vi "dNetOut_dOutH1.vi"(11 "OutH2":sgl[](array[numeric])) -> (3 "Output":sgl[](array[numeric]))   [LabVIEW 2020]
uses:
  <vilib>/rvi/Memory/Memory_Emulation/nirvimemoryFastEmulation.vi
  <vilib>/rvi/Memory/Memory_Emulation/nirvimemoryEmulation.vi
  <vilib>/rvi/Emulation/niFpgaEmulationIsFPGAContextNoSignature.vi
  <vilib>/rvi/DataTransferAndStorage/Container/Common/niFpgaContainerGetUniqueNameForEmu.vi
  <vilib>/rvi/Emulation/niFpgaProcessEmulError.vi
  <vilib>/rvi/Emulation/niFpgaSctlEmulationGetInTimedLoop.vi
  <vilib>/rvi/errors/nirviReportUnexpectedCaseInternalError (U32).vi
  <vilib>/rvi/DataTransferAndStorage/Container/XNode/niFpgaContainer.xnode
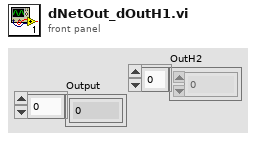
[diagram p1: front panel]
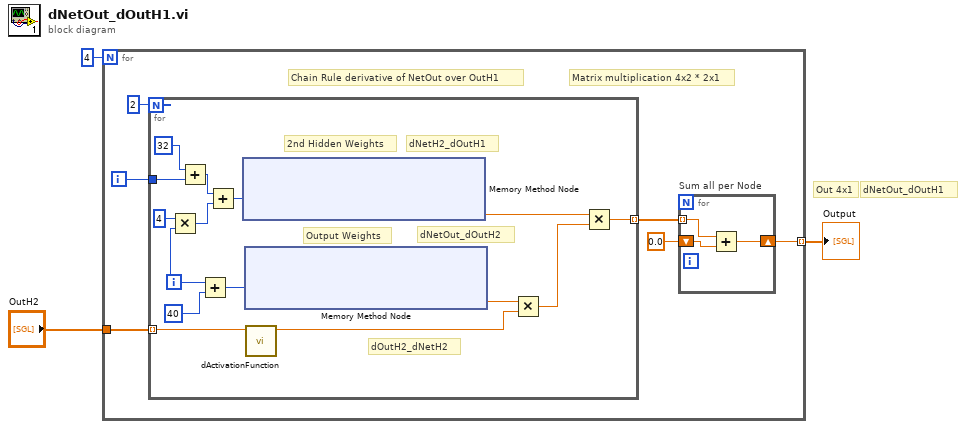
[diagram p0: block diagram]
diagram:
  # "dNetOut_dOutH1"
  # "Out 4x1"
  n1 = for {
    N: 4 -> [_]
    tunnel: [w7] -> w3 mode=indexing
    tunnel: "OutH2" -> [w5]
    i -> [w4]
    # "Matrix multiplication 4x2 * 2x1"
    # "Chain Rule derivative of NetOut over OutH1"
    n2 = for {
      N: 2 -> [_]
      tunnel: [w27] -> w6 mode=indexing
      tunnel: w5 -> [w20] mode=indexing
      tunnel: w4 -> [w13]
      i -> [w17]
      # "dNetH2_dOutH1"
      # "dNetOut_dOutH2"
      # "dOutH2_dNetH2"
      # "Output Weights"
      # "2nd Hidden Weights"
      n3 = Multiply(x=4, y=w17) -> (x*y=w18:i32)
      n4 = Add(x=32, y=w13) -> (x+y=w15:i32)
      n5 = Add(x=w17, y=40) -> (x+y=w24:i32)
      n6 = Add(x=w15, y=w18) -> (x+y=w23:i32)
      n7 = xnode ("Memory Method Node")("Address"=w23) -> ("Data"=w26:sgl)  [unwired: 1 in, 1 out]
      n8 = xnode ("Memory Method Node")("Address"=w24) -> ("Data"=w21:sgl)  [unwired: 1 in, 1 out]
      n9 = call "dActivationFunction.vi"("Output"=w20) -> ("f"=w19:sgl)  [unwired: 10 in]
      n10 = Multiply(x=w21, y=w19) -> (x*y=w22:sgl)
      n11 = Multiply(x=w26, y=w22) -> (x*y=w27:sgl)
    }
    n12 = for "Sum all per Node" {
      tunnel: w6 -> [w12] mode=indexing
      shift-right: [w10] -> w7
      shift-left: sgl 0.0 -> [w11]
      n13 = Add(x=w12, y=w11) -> (x+y=w10:sgl)
    }
  }
  "Output" <- w3
